vi "Close.vi"(8 "error in (no error)":errorcluster, 11 "EK-P4 in":refnum<class "EK-P4.lvclass">) -> (0 "error out":errorcluster, 3 "EK-P4 out":refnum<class "EK-P4.lvclass">)   [LabVIEW 2016, in "EK-P4.lvclass"]
doc: "Closes the connection to the EK-P4 sensirion board"
uses:
  EK-P4.lvclass
  EK-P4.lvclass/EK-P4.ctl
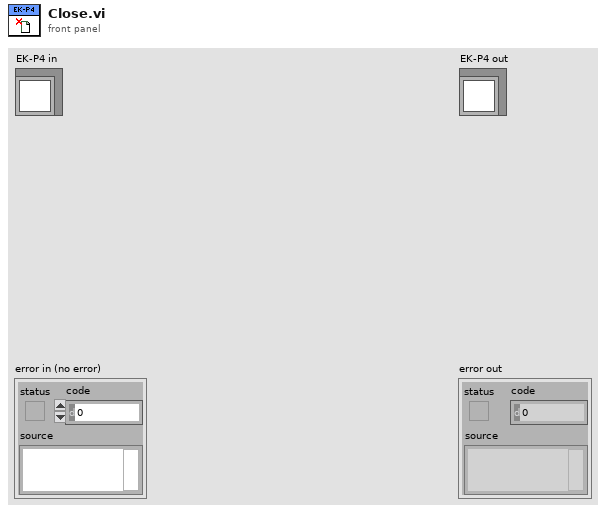
[diagram p1: front panel]
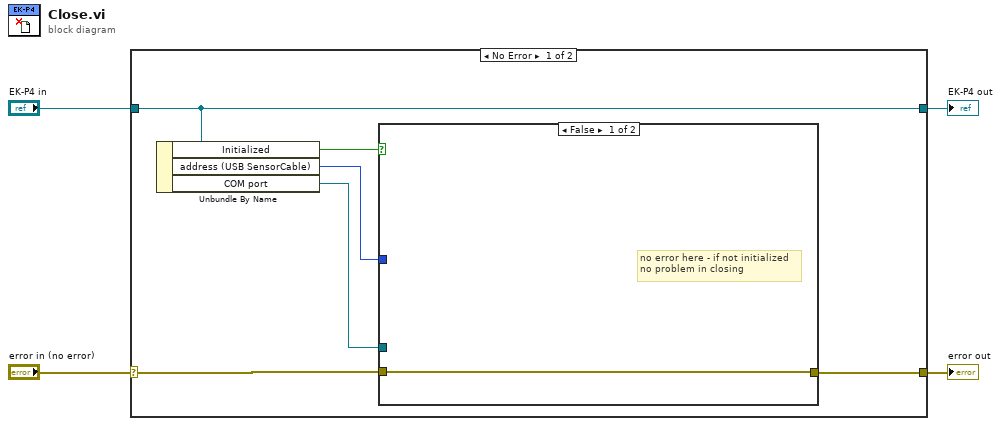
[diagram p0: block diagram]
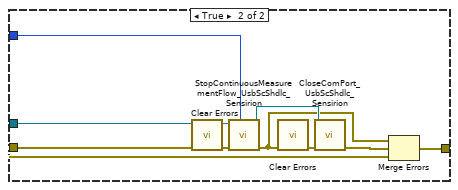
[diagram p2: hidden frame]
diagram:
  n1 = case shown="No Error" "error in (no error)" {
    selector: "error in (no error)" -> [w6 w22]
    tunnel: [w10 w22] -> w3
    tunnel: [w9 w21] -> w1
    tunnel: "EK-P4 in" -> [w9 w21]
    frame No Error {
      n2 = Unbundle By Name(w9) -> ("Initialized"=w5:bool, "address (USB SensorCable)"=w7:u8, "COM port"=w8:refnum<visa-resource-name>)
      n3 = case shown="False" w5 {
        tunnel: [w11 w15] -> w10
        tunnel: w8 -> [_ w14]
        tunnel: w7 -> [_ w13]
        tunnel: w6 -> [w11 w12]
        frame False {
          # "no error here - if not initialized\nno problem in closing"
        }
        frame True {
          n4 = call <vilib>:"Clear Errors.vi"("error in (no error)"=w12) -> ("error out"=w19:errorcluster)  [unwired: 5 in, 1 out]
          n5 = call "StopContinuousMeasurementFlow_UsbScShdlc_Sensirion.vi"("address"=w13, "error in (no error)"=w19, "COM port"=w14) -> ("error out"=w16:errorcluster, "COM port out"=w20:refnum<visa-resource-name>)  [unwired: 7 in]
          n6 = call <vilib>:"Clear Errors.vi"("error in (no error)"=w16) -> ("error out"=w18:errorcluster)  [unwired: 5 in, 1 out]
          n7 = call "CloseComPort_UsbScShdlc_Sensirion.vi"("error in (no error)"=w18, "COM port"=w20) -> ("error out"=w17:errorcluster)  [unwired: 9 in]
          n8 = Merge Errors(w16, w17, w12) -> (w15:errorcluster)
        }
      }
    }
    frame Error {
    }
  }
  "error out" <- w3
  "EK-P4 out" <- w1
